vi "Joystick_Ref_Num.vi"() -> (3 "Joystick":cluster{"Drive_Joystick":T1, "Imp_Joystick":T1})   [LabVIEW 2014]
uses:
  <vilib>/Rock Robotics/WPI/Joystick/WPI_JoystickDevRef.ctl
  <vilib>/Rock Robotics/WPI/Joystick/WPI_JoystickDeviceEnum.ctl
  <vilib>/Rock Robotics/WPI/Joystick/WPI_JoystickGetSetRefNum.vi
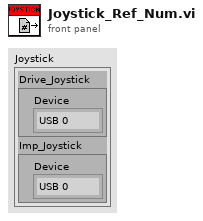
[diagram p1: front panel]
types:
  T1 = typedef "WPI_JoystickDevRef.ctl" = cluster{"Device":T2}
  T2 = typedef "WPI_JoystickDeviceEnum.ctl" = enum16{"USB 0", "USB 1", "USB 2", "USB 3", "USB 4", "USB 5"}
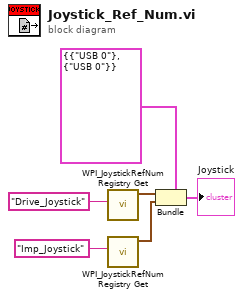
[diagram p0: block diagram]
diagram:
  n1 = call <vilib>:"WPI_JoystickRefNum Registry Get.vi"("refnum name"="Drive_Joystick") -> ("JoystickDevRef"=w3:T1)  [unwired: 1 in, 9 out]
  n2 = call <vilib>:"WPI_JoystickRefNum Registry Get.vi"("refnum name"="Imp_Joystick") -> ("JoystickDevRef"=w4:T1)  [unwired: 1 in, 9 out]
  n3 = Bundle(cluster=cluster{"Drive_Joystick":T1, "Imp_Joystick":T1} {"Drive_Joystick"={"Device"=enum."USB 0"}, "Imp_Joystick"={"Device"=enum."USB 0"}}, "Drive_Joystick"=w3, "Imp_Joystick"=w4) -> (→"Joystick":cluster{"Drive_Joystick":T1, "Imp_Joystick":T1})
